vi "solar_cfg Remove.vi"(0 "Config Refnum":refnum<data-value>, 1 "Section":string, 5 "Key":string, 11 "error in (no error)":errorcluster) -> (4 "dup Config Refnum":refnum<data-value>, 10 "Found?":bool, 15 "error out":errorcluster)   [LabVIEW 2018]
doc: "This VI removes a section or key from a configuration file. If Section & Key is found, then delete the key. If Section is found & Key is empty, then delete the section. Otherwise, do nothing."
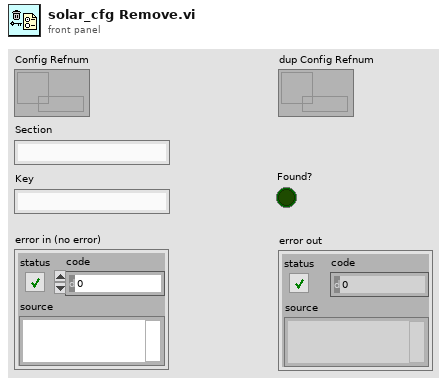
[diagram p1: front panel]
types:
  T1 = cluster{"Dirty":bool, "Semaphore":refnum<queue>, "Sections":cluster{"Section":string, "kvc":string[][]}[], "Path":path}
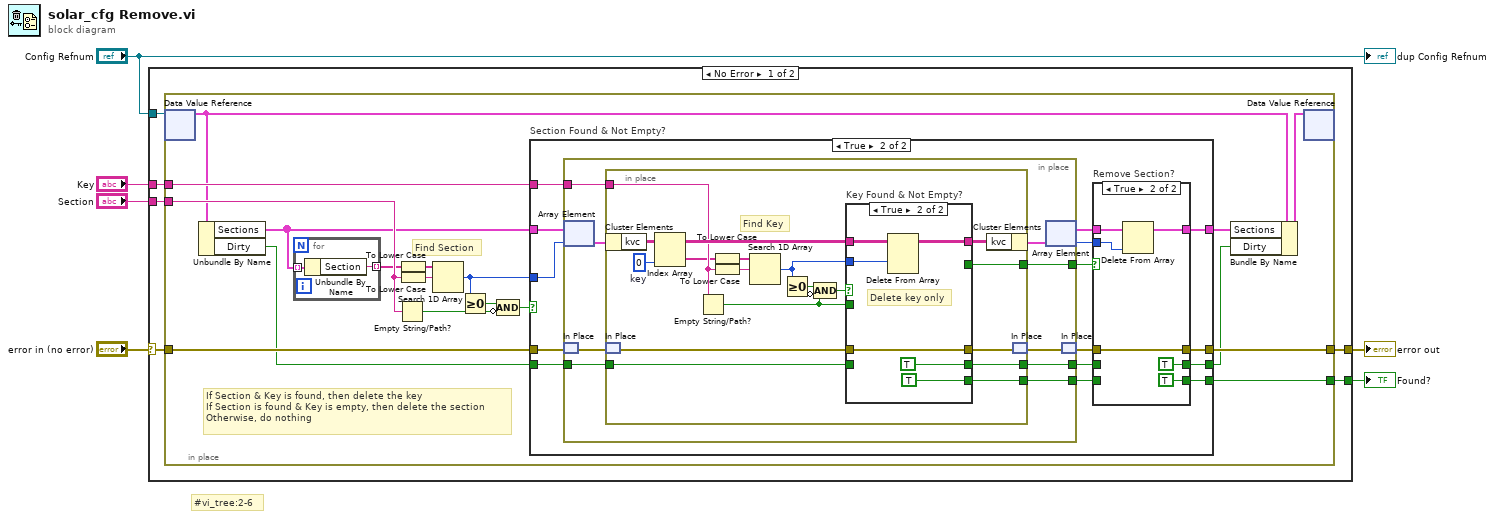
[diagram p0: block diagram]
diagram:
  # "#vi_tree:2-6"
  n1 = case shown="No Error" "error in (no error)" {
    selector: "error in (no error)" -> [w9 w97]
    tunnel: "Key" -> [w12 _]
    tunnel: [w8 w97] -> w4
    tunnel: "Section" -> [w10 _]
    tunnel: [w11 _] -> w2
    tunnel: "Config Refnum" -> [w7 _]
    frame No Error {
      n2 = in-place {
        in-place-border: w12 -> [w30]
        in-place-border: [w29] -> w11
        in-place-border: w10 -> [w28]
        in-place-border: w9 -> [w27]
        in-place-border: [w26] -> w8
        # "If Section & Key is found, then delete the key\nIf Section is found & Key is empty, then delete the section\nOtherwise, do nothing"
        # "Find Section"
        n3 = in-place-dvr #1(w7) -> (w14:T1)  [unwired: 1 out]
        n4 = Unbundle By Name(w14) -> ("Sections"=w18:cluster{"Section":string, "kvc":string[][]}[], "Dirty"=w15:bool)
        n5 = for {
          tunnel: w18 -> [w96] mode=indexing
          tunnel: [w95] -> w19 mode=indexing
          n6 = Unbundle By Name(w96) -> ("Section"=w95:string)
        }
        n7 = Empty String/Path?(string/path=w28) -> (empty?=w21:bool)
        n8 = To Lower Case(string=w19) -> (all lower case string=w24:string[])
        n9 = To Lower Case(string=w28) -> (all lower case string=w25:string)
        n10 = Search 1D Array(1D array=w24, element=w25) -> (index of element=w20:i32)  [unwired: 1 in]
        n11 = Greater Or Equal To 0?(x=w20) -> (x >= 0?=w23:bool)
        n12 = Compound Arithmetic op=AND(w23, invert w21) -> (w22:bool)
        n13 = case "Section Found & Not Empty?" shown="True" w22 {
          tunnel: w18 -> [w31 w47]
          tunnel: w27 -> [w33 w46]
          tunnel: w30 -> [_ w48]
          tunnel: [w33 w39] -> w26
          tunnel: [_ w34] -> w29
          tunnel: [w31 w41] -> w16
          tunnel: [w32 w37] -> w17
          tunnel: w20 -> [_ w45]
          tunnel: w15 -> [w32 w44]
          frame False {
          }
          frame True {
            n14 = in-place {
              in-place-border: w48 -> [w67]
              in-place-border: [w66] -> w35
              in-place-border: [w61] -> w36
              in-place-border: w44 -> [w60]
              in-place-border: [w59] -> w43
              n15 = in-place-array #2(w47, w45) -> (w65:cluster{"Section":string, "kvc":string[][]})
              n16 = in-place-match #3(w46) -> (w63:errorcluster)
              n17 = in-place {
                in-place-border: w67 -> [w75]
                in-place-border: [w81] -> w66
                in-place-border: [w76] -> w61
                in-place-border: w60 -> [w70]
                in-place-border: [w68] -> w59
                w84 = 0  # key
                # "Find Key"
                n18 = in-place-cluster #4(w65) -> ("kvc"=w80:string[][])
                n19 = in-place-match #5(w63) -> (w78:errorcluster)
                n20 = Index Array(array=w80, index (col)=w84) -> (element=w69:string[])  [unwired: 1 in]
                n21 = Empty String/Path?(string/path=w75) -> (empty?=w71:bool)
                n22 = To Lower Case(string=w69) -> (all lower case string=w83:string[])
                n23 = To Lower Case(string=w75) -> (all lower case string=w82:string)
                n24 = Search 1D Array(1D array=w83, element=w82) -> (index of element=w73:i32)  [unwired: 1 in]
                n25 = Greater Or Equal To 0?(x=w73) -> (x >= 0?=w74:bool)
                n26 = Compound Arithmetic op=AND(w74, invert w71) -> (w72:bool)
                n27 = case "Key Found & Not Empty?" shown="True" w72 {
                  tunnel: [w87 w93] -> w77
                  tunnel: w78 -> [w87 w93]
                  tunnel: w80 -> [w88 w91]
                  tunnel: [_ TRUE] -> w81
                  tunnel: [w88 w90] -> w79
                  tunnel: [w86 TRUE ("Write File")] -> w76
                  tunnel: w73 -> [_ w92]
                  tunnel: w71 -> [w85 _]
                  tunnel: w70 -> [w86 _]
                  tunnel: [w85 _] -> w68
                  frame False {
                    # "Key empty,\ndelete section"
                  }
                  frame True {
                    # "Delete key only"
                    n28 = Delete From Array(array=w91, index (row)=w92) -> (array with subset deleted=w90:string[][])  [unwired: 2 in, 1 out]
                  }
                }
                n29 = in-place-cluster #4("kvc"=w79) -> (w64:cluster{"Section":string, "kvc":string[][]})
                n30 = in-place-match #5(w77) -> (w62:errorcluster)
              }
              n31 = in-place-array #2(w64) -> (w42:cluster{"Section":string, "kvc":string[][]}[], w40:i32)
              n32 = in-place-match #3(w62) -> (w38:errorcluster)
            }
            n33 = case "Remove Section?" shown="True" w43 {
              tunnel: w42 -> [w52 w58]
              tunnel: [w52 w57] -> w41
              tunnel: w40 -> [_ w56]
              tunnel: [w51 w55] -> w39
              tunnel: w38 -> [w51 w55]
              tunnel: [w50 TRUE ("Write File")] -> w37
              tunnel: w36 -> [w50 _]
              tunnel: w35 -> [w49 _]
              tunnel: [w49 TRUE] -> w34
              frame False {
              }
              frame True {
                n34 = Delete From Array(array=w58, index=w56) -> (array with subset deleted=w57:cluster{"Section":string, "kvc":string[][]}[])  [unwired: 1 in, 1 out]
              }
            }
          }
        }
        n35 = Bundle By Name(cluster=w14, "Sections"=w16, "Dirty"=w17) -> (w13:T1)
        n36 = in-place-dvr #1(w13) -> ()  [unwired: 2 out]
      }
    }
    frame Error {
    }
  }
  "error out" <- w4
  "Found?" <- w2
  "dup Config Refnum" <- "Config Refnum"
